vi "ReadPhysicalParam.vi"(11 "堆物理参数文件路径":path) -> (0 "源项":sgl, 1 "中子寿命(s)":sgl, 2 "lamda":sgl[](array[numeric]), 3 "beta":sgl[](array[numeric]))   [LabVIEW 2020]
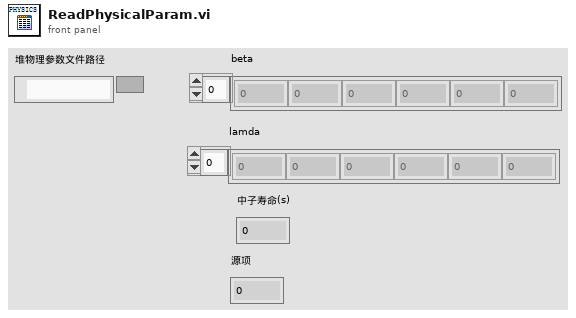
[diagram p1: front panel]
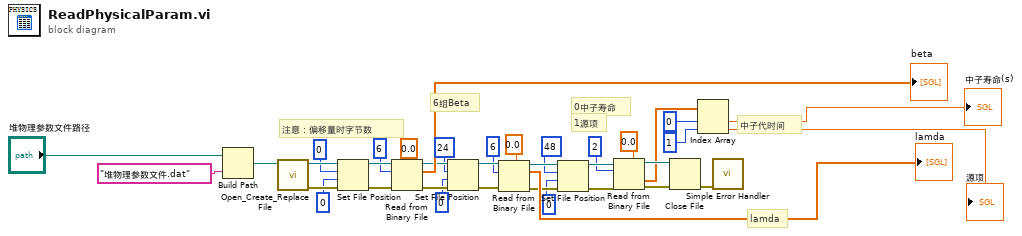
[diagram p0: block diagram]
diagram:
  # "注意：偏移量时字节数"
  # "0中子寿命"
  # "1源项"
  # "6组Beta"
  # "中子代时间"
  # "lamda"
  n1 = Build Path(base path="堆物理参数文件路径", name or relative path="堆物理参数文件.dat" ("string")) -> (appended path=w18:path)
  n2 = call <vilib>:"Open_Create_Replace File.vi"("file path"=w18) -> ("error out"=w33:errorcluster, "refnum"=w32:refnum<file>)  [unwired: 7 in, 2 out]
  n3 = Set File Position(offset (in bytes) (0)=0, refnum=w32, from (0:start)=0, error in=w33) -> (refnum out=w21:refnum<file>, error out=w22:errorcluster)
  n4 = Read from Binary File(5:sgl 0.0, 8:w22, 10:6, 11:w21) -> (0:w26:errorcluster, 2:→"beta":sgl[], 3:w25:refnum<file>)  [unwired: 2 in, 1 out]
  n5 = Set File Position(offset (in bytes) (0)=24, refnum=w25, from (0:start)=0, error in=w26) -> (refnum out=w23:refnum<file>, error out=w24:errorcluster)
  n6 = Read from Binary File(5:sgl 0.0, 8:w24, 10:6, 11:w23) -> (0:w28:errorcluster, 2:→"lamda":sgl[], 3:w27:refnum<file>)  [unwired: 2 in, 1 out]
  n7 = Set File Position(offset (in bytes) (0)=48, refnum=w27, from (0:start)=0, error in=w28) -> (refnum out=w19:refnum<file>, error out=w20:errorcluster)
  n8 = Read from Binary File(5:sgl 0.0, 8:w20, 10:2, 11:w19) -> (0:w30:errorcluster, 2:w10:sgl[], 3:w29:refnum<file>)  [unwired: 2 in, 1 out]
  n9 = Close File(refnum=w29, error in=w30) -> (error out=w31:errorcluster)  [unwired: 1 out]
  n10 = Index Array(array=w10, index #1=0, index #2=1) -> (element #1=→"中子寿命(s)":sgl, element #2=→"源项":sgl)
  n11 = call <vilib>:"Simple Error Handler.vi"("error in (no error)"=w31) -> ()  [unwired: 4 in, 5 out]
